vi "Load Configuration Keys Into Set.vi"(8 "error in (no error)":errorcluster, 11 "Path":path) -> (0 "error out":errorcluster, 2 "Sections and keys":T1, 3 "Path Out":path)   [LabVIEW 2019, in "Personalities Tool.lvlib"]
doc: "This VI reads the keys in a given configuration file and loads all of them in a variant as attributs, so we can index them easily."
uses:
  Personalities Tool.lvlib
  <vilib>/Utility/config.llb/NI_LVConfig.lvlib
  src robot/Classes/Configuration File/Configuration File.lvclass
  <vilib>/Utility/config.llb/Read Key (I32).vi
  <vilib>/Utility/config.llb/Read Key (Double).vi
  <vilib>/Utility/config.llb/Read Key (Boolean).vi
  <vilib>/Utility/config.llb/Read Key (Path).vi
  <vilib>/Utility/config.llb/Read Key (String).vi
  <vilib>/Utility/config.llb/Read Key (U32).vi
  Controls/Sections and keys.ctl
panel:
  out "Key, Value":variant
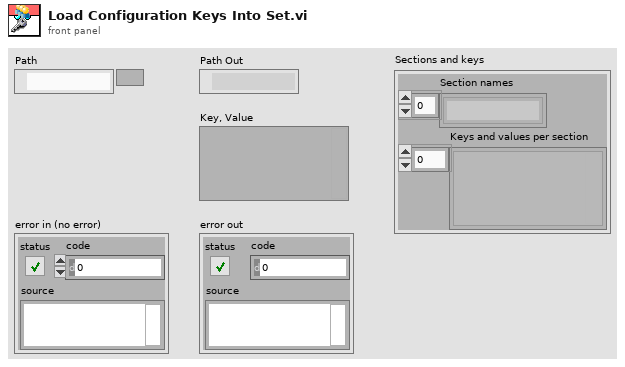
[diagram p1: front panel]
types:
  T1 = typedef "Personalities Tool.lvlib/Sections and keys.ctl" = cluster{"Section names":string[], "Keys and values per section":variant[]}
  T2 = typedef "NI_LVConfig.lvlib/Config Data RefNum.ctl" = refnum<k1>
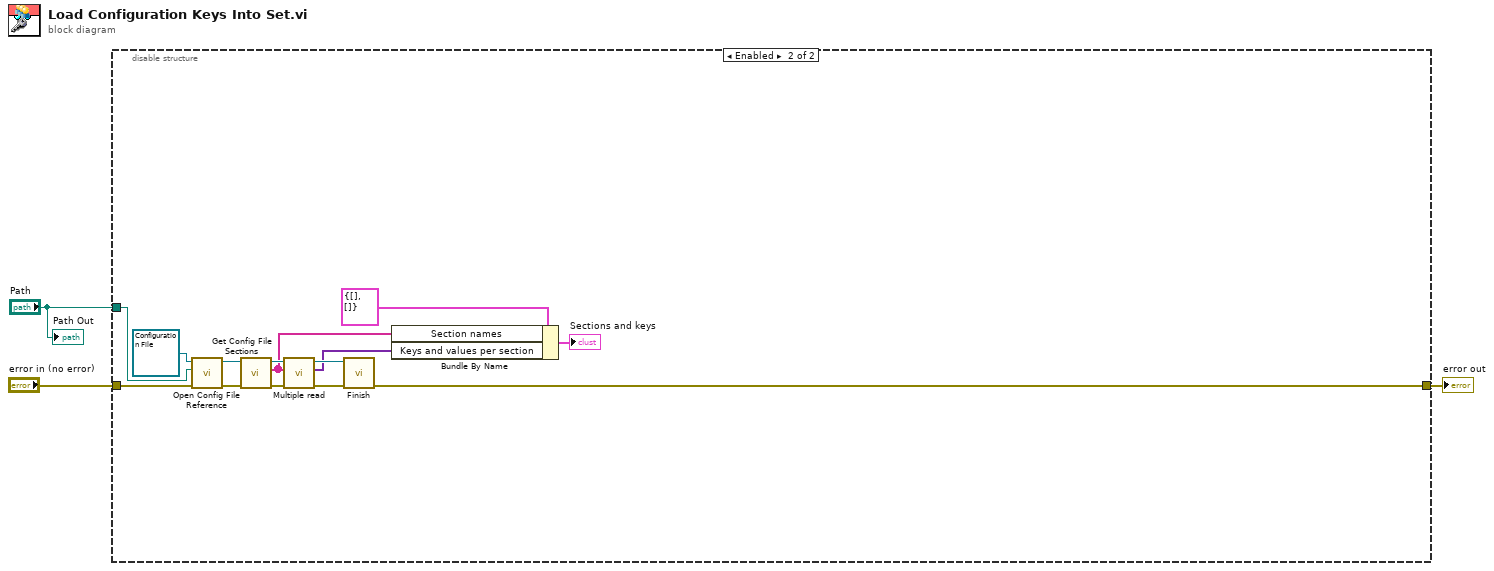
[diagram p0: block diagram]
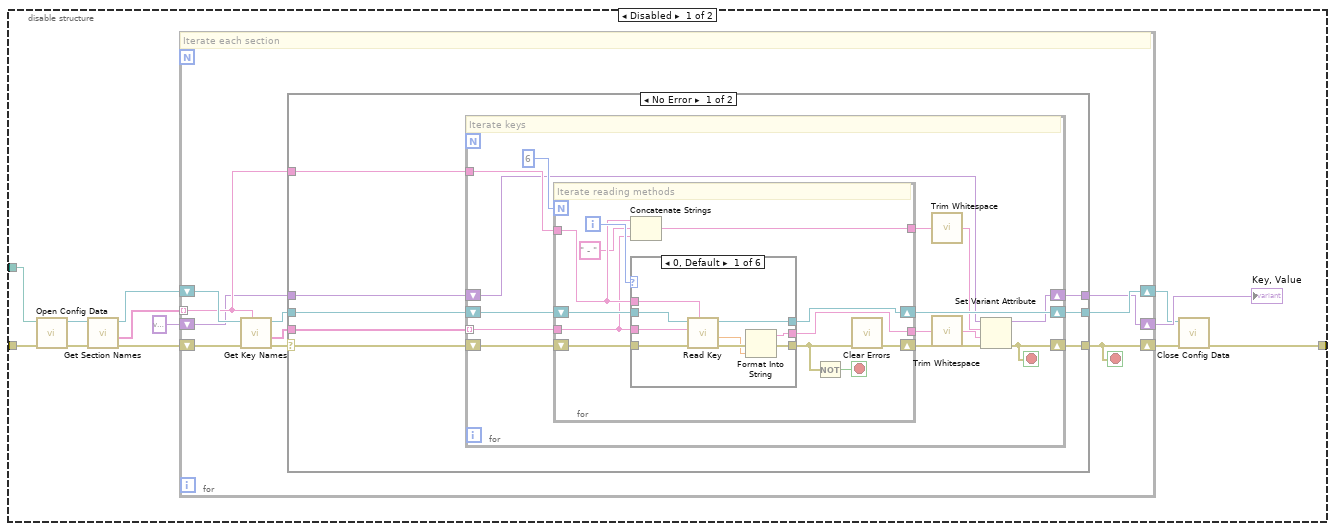
[diagram p2: hidden frame]
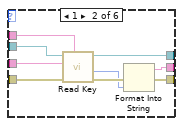
[diagram p3: hidden frame]
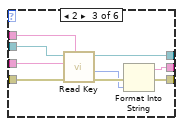
[diagram p4: hidden frame]
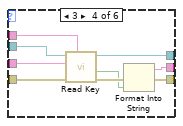
[diagram p5: hidden frame]
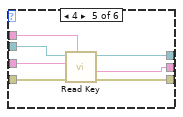
[diagram p6: hidden frame]
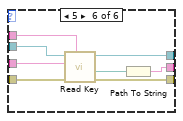
[diagram p7: hidden frame]
diagram:
  n1 = disable-structure shown="Enabled" {
    disable-tunnel: "Path" -> [w13 w121]
    disable-tunnel: [w12 w119] -> w3
    disable-tunnel: "error in (no error)" -> [w11 w122]
    frame Disabled {
      n2 = call <vilib>:"Open Config Data.vi"("error in (no error)"=w11, "configuration file path"=w13) -> ("error out"=w5:errorcluster, "refnum"=w4:T2)  [unwired: 7 in, 1 out]
      n3 = call <vilib>:"Get Section Names.vi"("error in (no error)"=w5, "refnum"=w4) -> ("error out"=w7:errorcluster, "section names"=w10:string[], "refnum out"=w6:T2)  [unwired: 7 in]
      n4 = for {
        shift-right: [w22] -> w8
        shift-left: w6 -> [w26]
        shift-right: [w21] -> w9
        shift-left: w7 -> [w25]
        tunnel: w10 -> [w19] mode=indexing
        shift-right: [w17] -> w16
        shift-left: variant -> [w18]
        stop <- w21 stop-if-true
        # "Iterate each section"
        n5 = call <vilib>:"Get Key Names.vi"("section"=w19, "error in (no error)"=w25, "refnum"=w26) -> ("error out"=w24:errorcluster, "key names"=w20:string[], "refnum out"=w23:T2)  [unwired: 5 in, 1 out]
        n6 = case shown="No Error" w24 {
          selector: w24 -> [w34 w113]
          tunnel: [w33 w113] -> w21
          tunnel: w23 -> [w32 w114]
          tunnel: [w31 w114] -> w22
          tunnel: w20 -> [w30 _]
          tunnel: w19 -> [w29 _]
          tunnel: w18 -> [w28 w112]
          tunnel: [w27 w112] -> w17
          frame No Error {
            n7 = for {
              tunnel: w30 -> [w45] mode=indexing
              shift-right: [w37] -> w33
              shift-left: w34 -> [w48]
              shift-right: [w46] -> w31
              shift-left: w32 -> [w47]
              tunnel: w29 -> [w44]
              shift-right: [w42] -> w27
              shift-left: w28 -> [w41]
              stop <- w37 stop-if-true
              # "Iterate keys"
              n8 = for {
                N: 6 -> [_]
                shift-right: [w54] -> w38
                shift-left: w48 -> [w60]
                shift-right: [w58] -> w46
                shift-left: w47 -> [w59]
                tunnel: w45 -> [w50]
                tunnel: w44 -> [w53]
                tunnel: [w51] -> w40
                tunnel: [w49] -> w39
                i -> [w56]
                stop <- w55 stop-if-true
                # "Iterate reading methods"
                n9 = Concatenate Strings(w53, " - " ("string"), w50) -> (w51:string)
                n10 = case shown="0, Default" w56 {
                  tunnel: w60 -> [w69 w78 w87 w96 w102 w111]
                  tunnel: w59 -> [w68 w77 w86 w95 w103 w110]
                  tunnel: [w67 w76 w85 w94 w100 w109] -> w58
                  tunnel: [w63 w72 w81 w90 w101 w104] -> w57
                  tunnel: w50 -> [w65 w74 w83 w92 w98 w108]
                  tunnel: w53 -> [w64 w73 w82 w91 w99 w107]
                  tunnel: [w61 w70 w79 w88 w97 w106] -> w49
                  frame 0, Default {
                    n11 = call-poly <vilib>:"Read Key.vi"("section"=w64, "error in (no error)"=w69, "key"=w65, "refnum"=w68) -> ("error out"=w66:errorcluster, "value"=w62:dbl, "refnum out"=w67:T2)  [unwired: 4 in, 1 out]
                    n12 = Format Into String(error in=w66, w62) -> (resulting string=w61:string, error out=w63:errorcluster)  [unwired: 2 in]
                  }
                  frame 1 {
                    n13 = call-poly <vilib>:"Read Key.vi"("section"=w73, "error in (no error)"=w78, "key"=w74, "refnum"=w77) -> ("error out"=w75:errorcluster, "value"=w71:i32, "refnum out"=w76:T2)  [unwired: 4 in, 1 out]
                    n14 = Format Into String(error in=w75, w71) -> (resulting string=w70:string, error out=w72:errorcluster)  [unwired: 2 in]
                  }
                  frame 2 {
                    n15 = call-poly <vilib>:"Read Key.vi"("section"=w82, "error in (no error)"=w87, "key"=w83, "refnum"=w86) -> ("error out"=w84:errorcluster, "value"=w80:u32, "refnum out"=w85:T2)  [unwired: 4 in, 1 out]
                    n16 = Format Into String(error in=w84, w80) -> (resulting string=w79:string, error out=w81:errorcluster)  [unwired: 2 in]
                  }
                  frame 3 {
                    n17 = call-poly <vilib>:"Read Key.vi"("section"=w91, "error in (no error)"=w96, "key"=w92, "refnum"=w95) -> ("error out"=w93:errorcluster, "value"=w89:bool, "refnum out"=w94:T2)  [unwired: 4 in, 1 out]
                    n18 = Format Into String(error in=w93, w89) -> (resulting string=w88:string, error out=w90:errorcluster)  [unwired: 2 in]
                  }
                  frame 4 {
                    n19 = call-poly <vilib>:"Read Key.vi"("section"=w99, "error in (no error)"=w102, "key"=w98, "refnum"=w103) -> ("error out"=w101:errorcluster, "value"=w97:string, "refnum out"=w100:T2)  [unwired: 4 in, 1 out]
                  }
                  frame 5 {
                    n20 = call-poly <vilib>:"Read Key.vi"("section"=w107, "error in (no error)"=w111, "key"=w108, "refnum"=w110) -> ("error out"=w104:errorcluster, "value"=w105:path, "refnum out"=w109:T2)  [unwired: 4 in, 1 out]
                    n21 = Path To String(path=w105) -> (string=w106:string)
                  }
                }
                n22 = Not(x=w57) -> (.not. x?=w55:bool)
                n23 = call <vilib>:"Clear Errors.vi"("error in (no error)"=w57) -> ("error out"=w54:errorcluster)  [unwired: 5 in, 1 out]
              }
              n24 = call <vilib>:"Trim Whitespace.vi"("string"=w40) -> ("trimmed string"=w36:string)  [unwired: 1 in]
              n25 = call <vilib>:"Trim Whitespace.vi"("string"=w39) -> ("trimmed string"=w35:string)  [unwired: 1 in]
              n26 = Set Variant Attribute(Variant=w41, name=w36, value=w35, error in=w38) -> (Variant out=w42:variant, error out=w37:errorcluster)  [unwired: 1 out]
            }
          }
          frame Error {
          }
        }
      }
      "Key, Value" <- w16
      n27 = call <vilib>:"Close Config Data.vi"("error in (no error)"=w9, "refnum"=w8) -> ("error out"=w12:errorcluster, "file path"=w14:path)  [unwired: 8 in]
    }
    frame Enabled {
      n28 = call "Open Config File Reference.vi"("error in (no error)"=w122, "appended path"=w121, "Configuration File in"=refnum<class "Configuration File.lvclass"> refnum) -> ("error out"=w128:errorcluster, "Configuration File out"=w127:refnum<class "Configuration File.lvclass">)  [unwired: 7 in]
      n29 = call-dynamic "Get Config File Sections.vi"("error in (no error)"=w128, "Configuration File in"=w127) -> ("error out"=w124:errorcluster, "Section names"=w116:string[], "Configuration File out"=w123:refnum<class "Configuration File.lvclass">)  [unwired: 7 in]
      n30 = call-dynamic "Multiple read.vi"("error in (no error)"=w124, "Section Names"=w116, "Configuration File in"=w123) -> ("error out"=w126:errorcluster, "Data Out"=w115:variant[], "Configuration File out"=w125:refnum<class "Configuration File.lvclass">)  [unwired: 5 in, 1 out]
      n31 = call-dynamic "Finish.vi"("error in (no error)"=w126, "Configuration File in"=w125) -> ("error out"=w119:errorcluster)  [unwired: 6 in, 3 out]
      n32 = Bundle By Name(cluster=T1 {"Section names"=[], "Keys and values per section"=[]} ("Sections and keys"), "Section names"=w116, "Keys and values per section"=w115) -> (→"Sections and keys":T1)
    }
  }
  "error out" <- w3
  "Path Out" <- "Path"
